vi "Clamp Upper.vi"(4 "Button":bool) -> (1 "Clamp State":T1)   [LabVIEW 2014]
uses:
  <vilib>/Rock Robotics/WPI/Solenoid/WPI_SolenoidValue.ctl
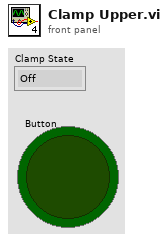
[diagram p1: front panel]
types:
  T1 = typedef "WPI_SolenoidValue.ctl" = enum16{"Off", "On", "Forward", "Reverse"}
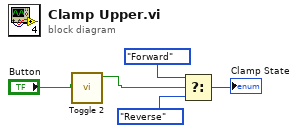
[diagram p0: block diagram]
diagram:
  n1 = call "Toggle 2.vi"("Input"="Button") -> ("Output"=w1:bool)  [unwired: 10 in]
  n2 = Select(t=WPI_SolenoidValue."Forward" ("Value"), s=w1, f=WPI_SolenoidValue."Reverse" ("Value")) -> (s? t:f=→"Clamp State":T1)
